vi "Remove Channel.vi"(8 "error in (no error)":errorcluster, 10 "Channel to remove":i32, 11 "Sequencer in":refnum<class "Sequencer.lvclass">) -> (0 "error out":errorcluster, 3 "Sequencer out":refnum<class "Sequencer.lvclass">)   [LabVIEW 2015, in "Sequencer.lvlib" / "Sequencer.lvclass"]
uses:
  Sequencer.lvclass
  <vilib>/ActorFramework/Stop Msg/Stop Msg.lvclass
  SequencerInfo.lvclass
  SequencerConfig.lvclass
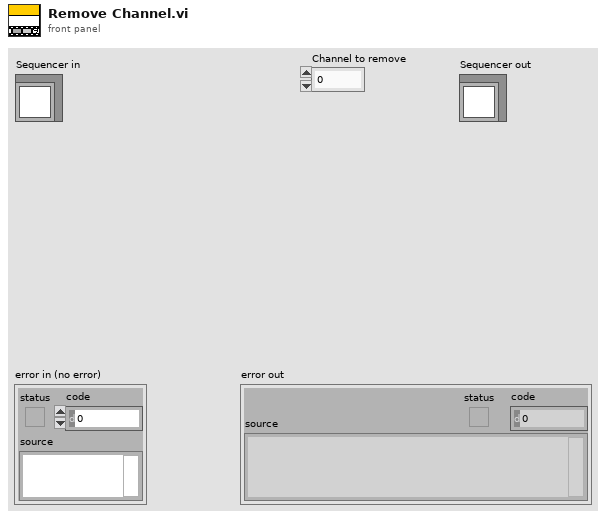
[diagram p1: front panel]
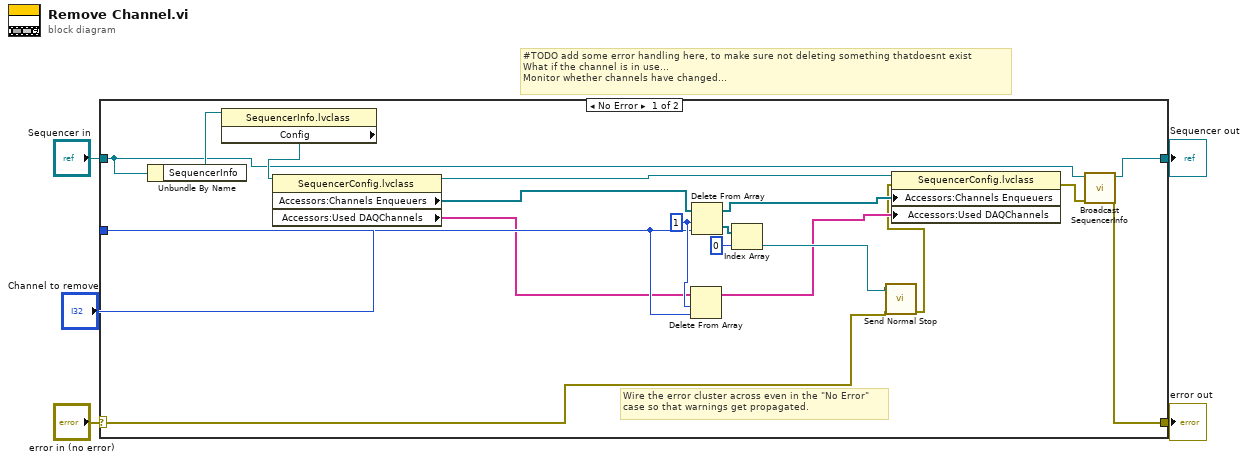
[diagram p0: block diagram]
diagram:
  # "#TODO add some error handling here, to make sure not deleting something thatdoesnt exist\nWhat if the channel is in use...\nMonitor whether channels have changed..."
  n1 = case shown="No Error" "error in (no error)" {
    selector: "error in (no error)" -> [w19 w25]
    tunnel: [w7 w25] -> w4
    tunnel: [w8 w24] -> w2
    tunnel: "Sequencer in" -> [w9 w24]
    tunnel: "Channel to remove" -> [w21 _]
    frame No Error {
      w22 = 1 ("length")
      # "Wire the error cluster across even in the \"No Error\"\ncase so that warnings get propagated."
      n2 = Unbundle By Name(w9) -> ("SequencerInfo"=w17:refnum<class "SequencerInfo.lvclass">)
      n3 = property class="SequencerInfo.lvclass"(reference=w17) -> ("Config"=w16:refnum<class "SequencerConfig.lvclass">)  [unwired: 1 in, 2 out]
      n4 = property class="SequencerConfig.lvclass"(reference=w16) -> (reference out=w11:refnum<class "SequencerConfig.lvclass">, "Accessors:Channels Enqueuers"=w15:refnum<class "Message Enqueuer.lvclass">[], "Accessors:Used DAQChannels"=w14:tag[])  [unwired: 1 in, 1 out]
      n5 = Delete From Array(array=w14, length=w22, index=w21) -> (array with subset deleted=w12:tag[])  [unwired: 1 out]
      n6 = Delete From Array(array=w15, length=w22, index=w21) -> (deleted portion=w23:refnum<class "Message Enqueuer.lvclass">[], array with subset deleted=w13:refnum<class "Message Enqueuer.lvclass">[])
      n7 = Index Array(array=w23, index=0) -> (element=w18:refnum<class "Message Enqueuer.lvclass">)
      n8 = call <vilib>:"Send Normal Stop.vi"("error in (no error)"=w19, "Message Enqueuer"=w18) -> ("error out"=w10:errorcluster)  [unwired: 9 in]
      n9 = property class="SequencerConfig.lvclass"(reference=w11, error in=w10, "Accessors:Channels Enqueuers"=w13, "Accessors:Used DAQChannels"=w12) -> (error out=w6:errorcluster)  [unwired: 1 out]
      n10 = call "Broadcast SequencerInfo.vi"("error in (no error)"=w6, "Sequencer in"=w9) -> ("error out"=w7:errorcluster, "Sequencer out"=w8:refnum<class "Sequencer.lvclass">)  [unwired: 8 in]
    }
    frame Error {
    }
  }
  "error out" <- w4
  "Sequencer out" <- w2
